vi "CRITICAL.vi"(6 "Message":string, 8 "error in":errorcluster) -> (0 "error out":errorcluster)   [LabVIEW 2024, in "hse-logger.lvlib"]
doc: "Logs a message and the content of the error-cluster, if \"error in\" is True.\nAn error on the \"error in\" terminal is cleared on the \"error out\" terminal.\n\n____\nHAMPEL SOFTWARE ENGINEERING v2.2.2 (2025-01-16 15:41)"
uses:
  <vilib>/Hampel Software Engineering/HSE Logger/hse-logger.lvlib
  <vilib>/Utility/error.llb/Error Cluster From Error Code.vi
  <vilib>/Hampel Software Engineering/HSE Logger/Logger/Logger.lvclass
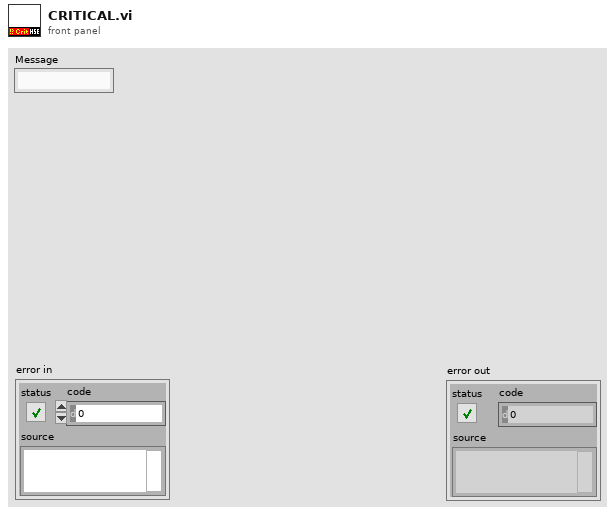
[diagram p1: front panel]
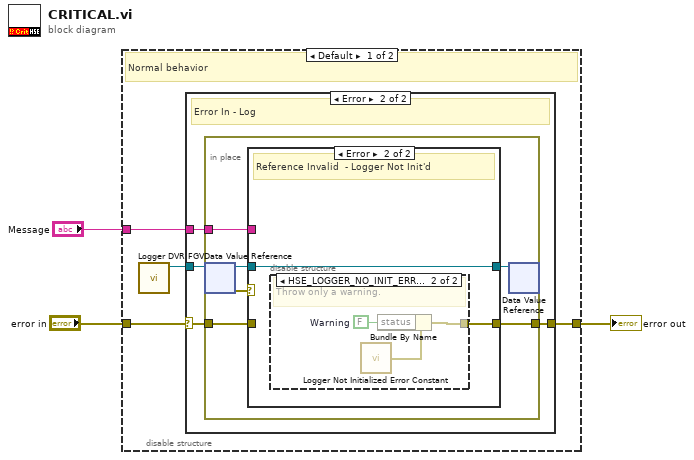
[diagram p0: block diagram]
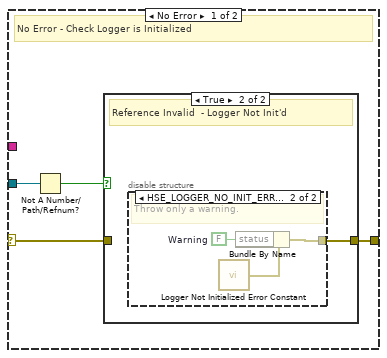
[diagram p2: hidden frame]
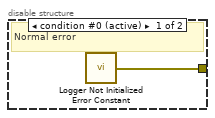
[diagram p4: hidden frame]
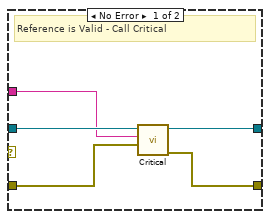
[diagram p5: hidden frame]
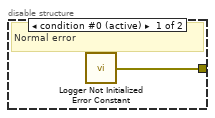
[diagram p6: hidden frame]
diagram:
  n1 = disable-structure shown="Default" {
    disable-tunnel: "error in" -> [w7 w39]
    disable-tunnel: [w6 w39] -> w2
    disable-tunnel: "Message" -> [w4 _]
    frame condition #0 (active) {
      # "Normal behavior"
      n2 = call <vilib>:"Logger DVR FGV.vi"() -> ("Logger DVR"=w5:refnum<data-value>)  [unwired: 10 in, 1 out]
      n3 = case shown="Error" w7 {
        selector: w7 -> [w9 w19]
        tunnel: w4 -> [_ w21]
        tunnel: [w8 w20] -> w6
        tunnel: w5 -> [w11 w18]
        frame No Error {
          # "No Error - Check Logger is Initialized"
          n4 = Not A Number/Path/Refnum?(number/path/refnum=w11) -> (NaN/Path/Refnum?=w10:bool)
          n5 = case shown="True" w10 {
            tunnel: w9 -> [w12 _]
            tunnel: [w12 w13] -> w8
            frame False {
              # "Reference is Valid - Do Nothing"
            }
            frame True {
              # "Reference Invalid  - Logger Not Init'd"
              n6 = disable-structure shown="HSE_LOGGER_NO_INIT_ERROR==True" {
                disable-tunnel: [w14 w16] -> w13
                frame condition #0 (active) {
                  # "Normal error"
                  n7 = call <vilib>:"Logger Not Initialized Error Constant.vi"() -> ("Logger Not Initialized Error"=w14:errorcluster)
                }
                frame condition #1 {
                  w15 = FALSE  # Warning
                  # "Throw only a warning."
                  n8 = call <vilib>:"Logger Not Initialized Error Constant.vi"() -> ("Logger Not Initialized Error"=w17:errorcluster)
                  n9 = Bundle By Name(cluster=w17, "status"=w15) -> (w16:errorcluster)
                }
              }
            }
          }
        }
        frame Error {
          # "Error In - Log"
          n10 = in-place {
            in-place-border: w21 -> [w26]
            in-place-border: [w25] -> w20
            in-place-border: w19 -> [w22]
            n11 = in-place-dvr #1(w18) -> (w27:refnum<class "Logger.lvclass">, w23:errorcluster)
            n12 = case shown="Error" w23 {
              tunnel: w27 -> [w32 w34]
              tunnel: w26 -> [w31 _]
              tunnel: [w30 w33] -> w25
              tunnel: [w29 w34] -> w24
              tunnel: w22 -> [w28 _]
              frame No Error {
                # "Reference is Valid - Call Critical"
                n13 = call-dynamic "Critical.vi"("Error to Log"=w28, "Message"=w31, "Logger in"=w32) -> ("error out"=w30:errorcluster, "Logger out"=w29:refnum<class "Logger.lvclass">)  [unwired: 7 in]
              }
              frame Error {
                # "Reference Invalid  - Logger Not Init'd"
                n14 = disable-structure shown="HSE_LOGGER_NO_INIT_ERROR==True" {
                  disable-tunnel: [w35 w37] -> w33
                  frame condition #0 (active) {
                    # "Normal error"
                    n15 = call <vilib>:"Logger Not Initialized Error Constant.vi"() -> ("Logger Not Initialized Error"=w35:errorcluster)
                  }
                  frame condition #1 {
                    w36 = FALSE  # Warning
                    # "Throw only a warning."
                    n16 = call <vilib>:"Logger Not Initialized Error Constant.vi"() -> ("Logger Not Initialized Error"=w38:errorcluster)
                    n17 = Bundle By Name(cluster=w38, "status"=w36) -> (w37:errorcluster)
                  }
                }
              }
            }
            n18 = in-place-dvr #1(w24) -> ()  [unwired: 2 out]
          }
        }
      }
    }
    frame condition #1 {
      # "Logging disabled"
    }
  }
  "error out" <- w2
